vi "GetFrontPanel.vi"(8 "Error In":errorcluster, 11 "object in":refnum<class "Mockup_QualificationScreen.lvclass">) -> (0 "Error Out":errorcluster, 2 "FrontPanel":refnum<class "FrontPanelControl.lvclass">, 3 "object out":refnum<class "Mockup_QualificationScreen.lvclass">)   [LabVIEW 2021, in "Mockup_QualificationScreen.lvclass"]
doc: "Retrieve the FrontPanelControl for controlling the state of the user interface front panel"
uses:
  Mockup_QualificationScreen.lvclass
  .Externals/Library_UserInterface_FrontPanelControl/FrontPanelControl/FrontPanelControl.lvclass
  Mockup_QualificationScreen.lvclass/Mockup_QualificationScreen.ctl
  <vilib>/Analysis/NI_AALBase.lvlib
panel:
  out "Histogram Graph":T1(graph)
  out "Image":picture
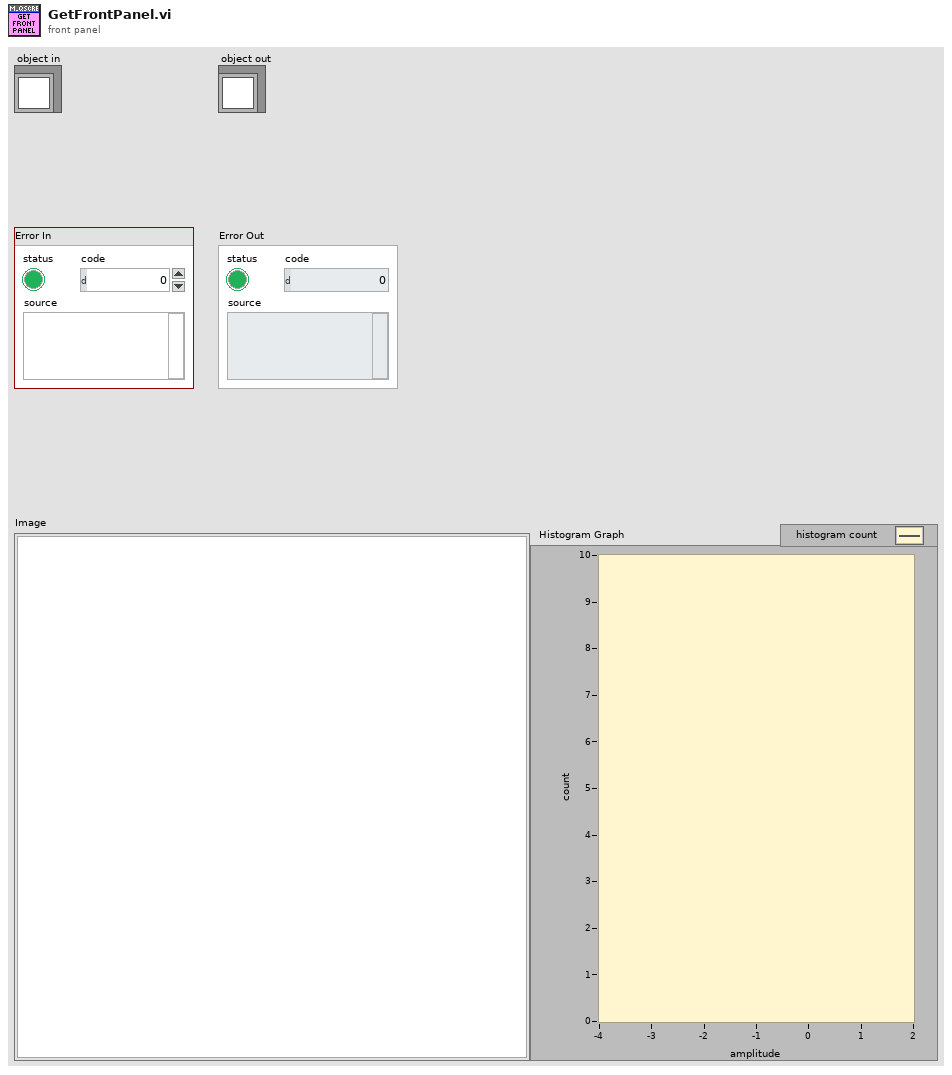
[diagram p1: front panel]
types:
  T1 = cluster{"X Values":dbl[], "Histogram: h(x)":i32[]}
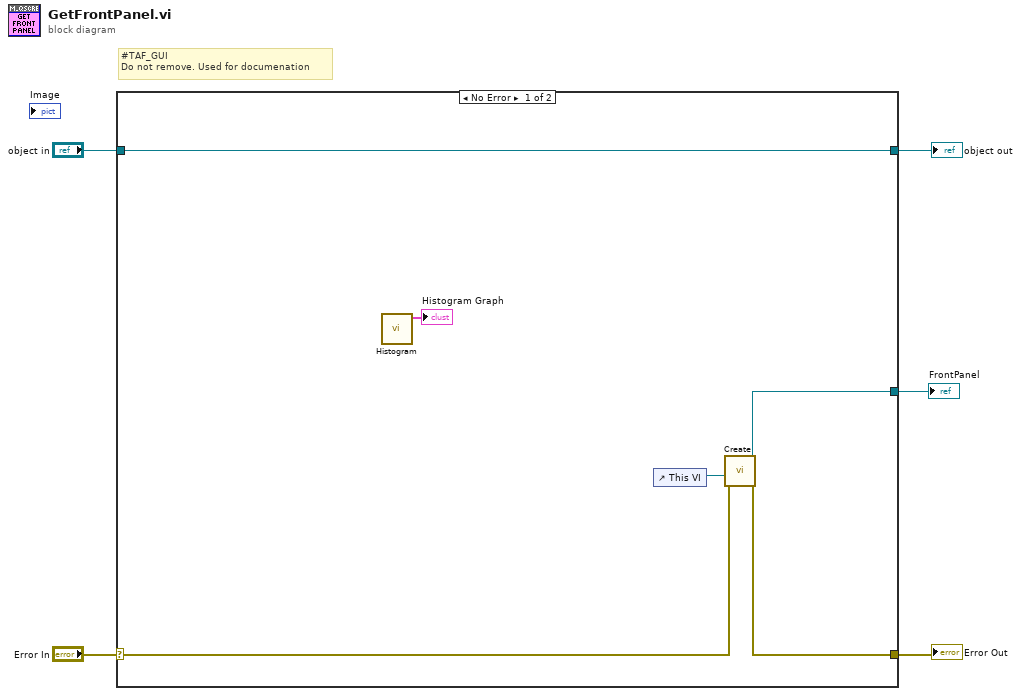
[diagram p0: block diagram]
diagram:
  # "#TAF_GUI\nDo not remove. Used for documenation"
  n1 = case shown="No Error" "Error In" {
    selector: "Error In" -> [w8 w13]
    tunnel: [w7 w13] -> w4
    tunnel: [w11 w12] -> w2
    tunnel: "object in" -> [w11 w12]
    tunnel: [w6 _] -> w1
    frame No Error {
      n2 = call <vilib>:"Histogram.vi"() -> ("Histogram Graph"=→"Histogram Graph":T1)  [unwired: 8 in, 3 out]
      n3 = control-ref of="This VI"() -> (w9:refnum<vi>)
      n4 = call "Create.vi"("ErrorIn"=w8, "VIRef"=w9) -> ("ErrorOut"=w7:errorcluster, "ObjectOut"=w6:refnum<class "FrontPanelControl.lvclass">)  [unwired: 8 in]
    }
    frame Error {
    }
  }
  "Error Out" <- w4
  "object out" <- w2
  "FrontPanel" <- w1
